vi "CRYextision level DIN.vi"(0 "extition level":dbl[](array[numeric])) -> (7 "LE":dbl[](array[numeric]), 9 "Ti":dbl[](array[numeric]))   [LabVIEW 2013]
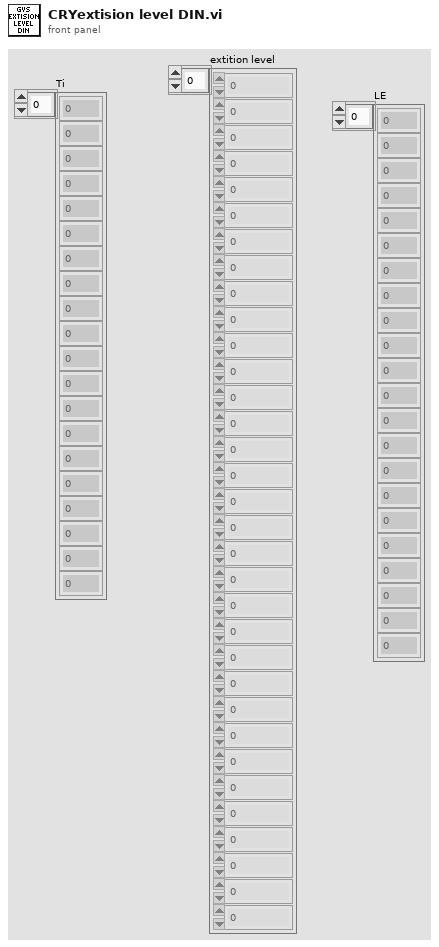
[diagram p1: front panel]
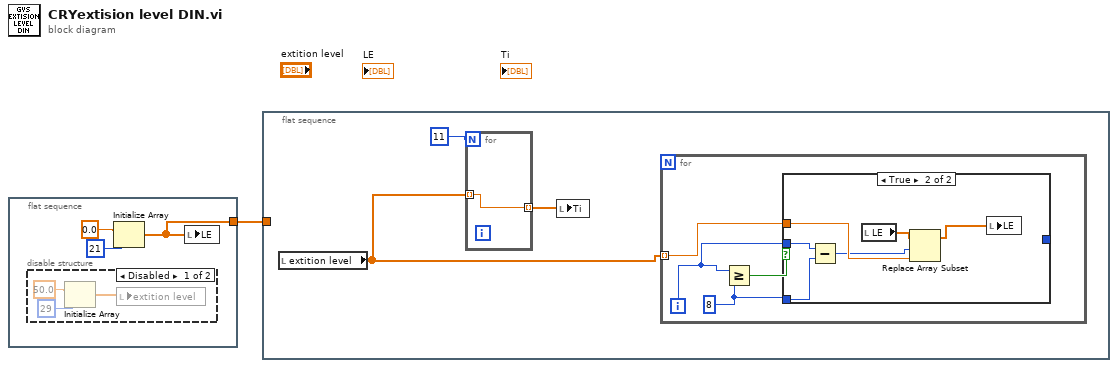
[diagram p0: block diagram]
diagram:
  n1 = flat-sequence {
    tunnel: [w2] -> w1
    frame #0 {
      n2 = disable-structure shown="Disabled" {
        frame Disabled {
          n3 = Initialize Array(50.0, 29) -> (w5:dbl[])
          n4 = local write "extition level"(w5) -> ()
        }
        frame Enabled {
        }
      }
      n5 = Initialize Array(0.0, 21) -> (w2:dbl[])
      n6 = local write "LE"(w2) -> ()
    }
  }
  n7 = flat-sequence {
    tunnel: w1 -> [_]
    frame #0 {
      n8 = local read "extition level"() -> (w8:dbl[])
      n9 = for {
        N: 11 -> [_]
        tunnel: [w22] -> w9 mode=indexing
        tunnel: w8 -> [w22] mode=indexing
      }
      n10 = local write "Ti"(w9) -> ()
      n11 = for {
        tunnel: w8 -> [w11] mode=indexing
        i -> [w13]
        w12 = 8
        n12 = Greater Or Equal?(x=w13, y=w12) -> (x >= y?=w14:bool)
        n13 = case shown="True" w14 {
          tunnel: w13 -> [w15 w21]
          tunnel: w12 -> [_ w20]
          tunnel: w11 -> [_ w18]
          tunnel: [w15 _] -> _
          frame False {
          }
          frame True {
            n14 = Subtract(x=w21, y=w20) -> (x-y=w17:i32)
            n15 = local read "LE"() -> (w19:dbl[])
            n16 = Replace Array Subset(array=w19, new element=w18, index=w17) -> (w16:dbl[])
            n17 = local write "LE"(w16) -> ()
          }
        }
      }
    }
  }
